vi "FTW-TransferClient-Download.vi"(0 "TransferClient.dotNET":refnum<class "FTW-TransferClient-dotNET.lvclass">, 11 "error in":errorcluster) -> (4 "TransferClient.dotNET out":refnum<class "FTW-TransferClient-dotNET.lvclass">, 6 "Data":string, 8 "Download Time":u32 format="%06dmsec", 15 "error out":errorcluster)   [LabVIEW 2014, in "FTW-TransferClient-dotNET.lvclass"]
uses:
  FTW-TransferClient-dotNET.lvclass
  FTW-TransferClient-dotNET.lvclass/FTW-TransferClient-dotNET.ctl
panel:
  # "Inputs"
  # "Outputs"
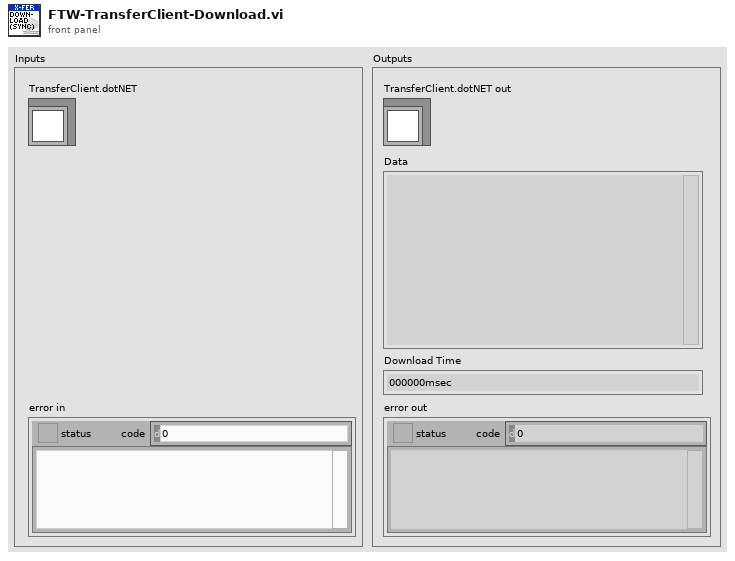
[diagram p1: front panel]
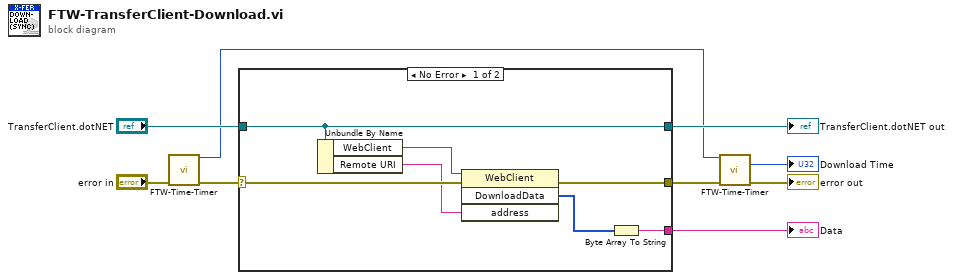
[diagram p0: block diagram]
diagram:
  n1 = call "FTW-Time-Timer.vi"("error in"="error in") -> ("Current Tick Count"=w2:u32, "error out"=w5:errorcluster)  [unwired: 12 in, 1 out]
  n2 = case shown="No Error" w5 {
    selector: w5 -> [w12 w17]
    tunnel: "TransferClient.dotNET" -> [w11 w18]
    tunnel: [w15 _] -> w8
    tunnel: [w14 w17] -> w3
    tunnel: [w11 w18] -> w7
    frame No Error {
      n3 = Unbundle By Name(w11) -> ("WebClient"=w13:refnum<k24>, "Remote URI"=w10:string)
      n4 = invoke class="WebClient" method="DownloadData"(reference=w13, error in=w12, "address"=w10) -> (error out=w14:errorcluster, "DownloadData"=w16:u8[])  [unwired: 1 in, 2 out]
      n5 = Byte Array To String(unsigned byte array=w16) -> (string=w15:string)
    }
    frame Error {
    }
  }
  "TransferClient.dotNET out" <- w7
  "Data" <- w8
  n6 = call "FTW-Time-Timer.vi"("Initial Tick Count"=w2, "error in"=w3) -> ("Elapsed Time"=→"Download Time":u32, "error out"=→"error out":errorcluster)  [unwired: 11 in, 1 out]
